vi "Keyed sort.vi"(2 "Re cal.[]":dbl[](array[numeric]), 3 "X cal.[]":dbl[](array[numeric])) -> (0 "Re cal. keyed sorted[]":dbl[](array[numeric]), 1 "X cal. sorted[]":dbl[](array[numeric]))   [LabVIEW 2020]
doc: "Sort X in ascending order and its corresponding Re values.\nPN 05-NOV-23."
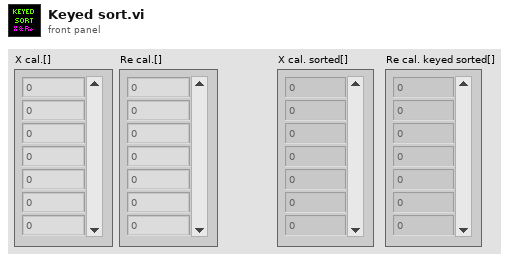
[diagram p1: front panel]
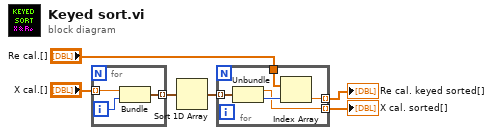
[diagram p0: block diagram]
diagram:
  n1 = for {
    tunnel: [w8] -> w5 mode=indexing
    tunnel: "X cal.[]" -> [w7] mode=indexing
    i -> [w9]
    n2 = Bundle("Numeric"=w7, w9) -> (w8:cluster{"Numeric":dbl, i32})  [unwired: 1 in]
  }
  n3 = Sort 1D Array(array=w5) -> (sorted array=w6:cluster{"Numeric":dbl, i32}[])
  n4 = for {
    tunnel: w6 -> [w14] mode=indexing
    tunnel: "Re cal.[]" -> [w12]
    tunnel: [w11] -> w1 mode=indexing
    tunnel: [w10] -> w2 mode=indexing
    n5 = Unbundle(w14) -> ("Numeric"=w10:dbl, w13:i32)
    n6 = Index Array(array=w12, index=w13) -> (element=w11:dbl)
  }
  "X cal. sorted[]" <- w2
  "Re cal. keyed sorted[]" <- w1
